vi "HTTPS Server Test with BIO & TCPIP Nodes.vi"() -> ()   [LabVIEW 2013]
uses:
  SSL_Lib/SSL-Lib/Library Paths.ctl
  SSL_Lib/SSL/SSL_Mode.ctl
  SSL_Lib/SSL-Lib/SSL-Lib.lvclass
  SSL_Lib/SSL-Context/SSL-Context.lvclass
  SSL_Lib/SSL/SSL.lvclass
  SSL_Lib/BIO/BIO.lvclass
panel:
  out "Read bytes":string
  out "Numeric":i32
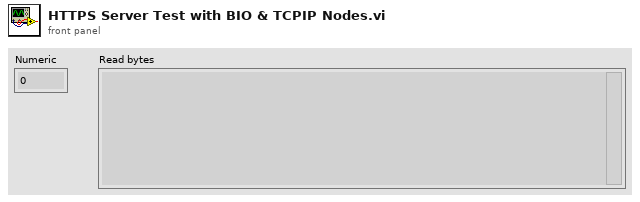
[diagram p1: front panel]
types:
  T1 = typedef "SSL_Lib.lvlib/SSL.lvclass/SSL_Mode.ctl" = i32
  T2 = typedef "SSL_Lib.lvlib/SSL-Lib.lvclass/Library Paths.ctl" = cluster{"SSL Library Path":path, "Crypto Library Path":path}
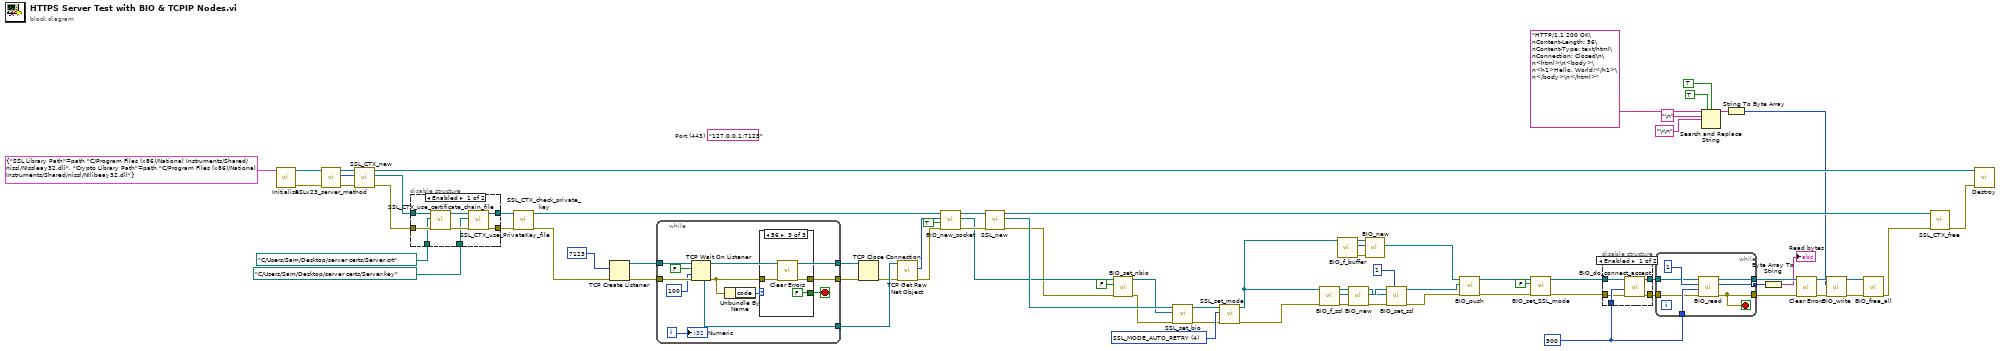
[diagram p0: block diagram]
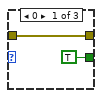
[diagram p3: hidden frame]
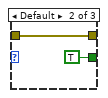
[diagram p4: hidden frame]
diagram:
  w49 = u32 500 ("Timeout (10000ms)")
  (unwired) "127.0.0.1:7123"  # Port (443)
  w63 = T1 4 items=["None"=0, "SSL_MODE_ENABLE_PARTIAL_WRITE"=1, "SSL_MODE_ACCEPT_MOVING_WRITE_BUFFER"=2, "SSL_MODE_AUTO_RETRY"=4, "SSL_MODE_RELEASE_BUFFERS"=16, "SSL_MODE_SEND_FALLBACK_SCSV"=128] ("Mode")
  n1 = call "Initialise.vi"("Library Paths"=T2 {"SSL Library Path"=path "C:/Program Files (x86)/National Instruments/Shared/nissl/NIssleay32.dll", "Crypto Library Path"=path "C:/Program Files (x86)/National Instruments/Shared/nissl/NIlibeay32.dll"}) -> ("error out"=w72:errorcluster, "SSL-Lib out"=w76:refnum<class "SSL-Lib.lvclass">)  [unwired: 9 in]
  n2 = call "SSLv23_server_method.vi"("error in (no error)"=w72, "SSL-Lib in"=w76) -> ("error out"=w70:errorcluster, "*SSL_Method"=w75:u64, "SSL-Lib out"=w74:refnum<class "SSL-Lib.lvclass">)  [unwired: 7 in]
  n3 = call "SSL_CTX_new.vi"("error in (no error)"=w70, "*SSL_Method"=w75, "SSL-Lib in"=w74) -> ("error out"=w69:errorcluster, "SSL-Context out"=w68:refnum<class "SSL-Context.lvclass">, "SSL-Lib out"=w62:refnum<class "SSL-Lib.lvclass">)  [unwired: 6 in]
  n4 = disable-structure shown="Enabled" {
    disable-tunnel: w69 -> [w82 w85]
    disable-tunnel: w68 -> [w81 w86]
    disable-tunnel: [w80 w85] -> w67
    disable-tunnel: [w79 w86] -> w66
    disable-tunnel: path "C:/Users/Sam/Desktop/server certs/Server.crt" -> [w78 _]
    disable-tunnel: path "C:/Users/Sam/Desktop/server certs/Server.key" -> [w77 _]
    frame Enabled {
      n5 = call "SSL_CTX_use_certificate_chain_file.vi"("error in (no error)"=w82, "Certificate Chain File"=w78, "SSL-Context in"=w81) -> ("error out"=w84:errorcluster, "SSL-Context out"=w83:refnum<class "SSL-Context.lvclass">)  [unwired: 7 in]
      n6 = call "SSL_CTX_use_PrivateKey_file.vi"("error in (no error)"=w84, "PrivateKey File"=w77, "SSL-Context in"=w83) -> ("error out"=w80:errorcluster, "SSL-Context out"=w79:refnum<class "SSL-Context.lvclass">)  [unwired: 7 in]
    }
    frame Disabled {
    }
  }
  n7 = call "SSL_CTX_check_private_key.vi"("error in (no error)"=w67, "SSL-Context in"=w66) -> ("error out"=w54:errorcluster, "SSL-Context out"=w43:refnum<class "SSL-Context.lvclass">)  [unwired: 8 in]
  n8 = TCP Create Listener(8:w54, 10:u16 7123 ("port")) -> (0:w60:errorcluster, 3:w59:refnum<k5>)  [unwired: 3 in, 1 out]
  n9 = while {
    tunnel: w60 -> [w97]
    tunnel: w59 -> [w96]
    tunnel: [w95] -> w58
    tunnel: [w91] -> w57
    tunnel: [w94] -> w56
    i -> [w87]
    stop <- w90 stop-if-true
    n10 = TCP Wait On Listener(8:w97, 9:100 ("timeout ms (wait forever: -1)"), 10:FALSE ("resolve remote address (T)"), 11:w96) -> (0:w92:errorcluster, 3:w95:refnum<k5>, 4:w94:refnum<k5>)  [unwired: 2 out]
    n11 = Unbundle By Name(w92) -> ("code"=w93:i32)
    n12 = case shown="56" w93 {
      tunnel: w92 -> [w99 w101 w104]
      tunnel: [w99 w101 w103] -> w91
      tunnel: [TRUE TRUE FALSE] -> w90
      frame 0 {
      }
      frame Default {
      }
      frame 56 {
        n13 = call <vilib>:"Clear Errors.vi"("error in (no error)"=w104) -> ("error out"=w103:errorcluster)  [unwired: 6 in]
      }
    }
    "Numeric" <- w87
  }
  n14 = TCP Close Connection(connection ID=w58, error in (no error)=w57) -> (error out=w55:errorcluster)  [unwired: 1 in, 1 out]
  n15 = call <vilib>:"TCP Get Raw Net Object.vi"("error in (no error)"=w55, "connection ID"=w56) -> ("error out"=w46:errorcluster, "raw net object"=w45:u64)  [unwired: 7 in, 1 out]
  n16 = call "BIO_new_socket.vi"("error in (no error)"=w46, "Close on free? (T)"=TRUE, "fd"=w45, "SSL-Context in"=w43) -> ("error out"=w42:errorcluster, "Socket BIO out"=w39:refnum<class "BIO.lvclass">, "SSL-Context out"=w41:refnum<class "SSL-Context.lvclass">)  [unwired: 5 in]
  n17 = call "SSL_new.vi"("error in (no error)"=w42, "SSL-Context in"=w41) -> ("error out"=w36:errorcluster, "SSL out"=w40:refnum<class "SSL.lvclass">, "SSL-Context out"=w53:refnum<class "SSL-Context.lvclass">)  [unwired: 7 in]
  n18 = call "BIO_set_nbio.vi"("error in (no error)"=w36, "Non-Blocking?"=FALSE, "BIO in"=w39) -> ("error out"=w35:errorcluster, "BIO out"=w37:refnum<class "BIO.lvclass">)  [unwired: 7 in]
  n19 = call "SSL_set_bio.vi"("error in (no error)"=w35, "BIO"=w37, "SSL in"=w40) -> ("error out"=w34:errorcluster, "SSL out"=w38:refnum<class "SSL.lvclass">)  [unwired: 7 in]
  n20 = call "SSL_set_mode.vi"("error in (no error)"=w34, "Mode"=w63, "SSL in"=w38) -> ("error out"=w25:errorcluster, "SSL out"=w18:refnum<class "SSL.lvclass">)  [unwired: 7 in]
  n21 = call "BIO_f_ssl.vi"("error in (no error)"=w25, "SSL-Lib in"=w18) -> ("error out"=w30:errorcluster, "*BIO_Method"=w28:u64, "SSL-Lib out"=w29:refnum<class "SSL.lvclass">)  [unwired: 7 in]
  n22 = call "BIO_f_buffer.vi"("SSL-Lib in"=w18) -> ("error out"=w33:errorcluster, "*BIO_Method"=w31:u64, "SSL-Lib out"=w32:refnum<class "SSL.lvclass">)  [unwired: 8 in]
  n23 = call "BIO_new.vi"("error in (no error)"=w30, "*BIO_method"=w28, "SSL-Lib in"=w29) -> ("error out"=w27:errorcluster, "BIO out"=w26:refnum<class "BIO.lvclass">, "SSL-Lib out"=w24:refnum<class "SSL.lvclass">)  [unwired: 6 in]
  n24 = call "BIO_new.vi"("error in (no error)"=w33, "*BIO_method"=w31, "SSL-Lib in"=w32) -> ("BIO out"=w22:refnum<class "BIO.lvclass">)  [unwired: 6 in, 2 out]
  n25 = call "BIO_set_ssl.vi"("close flag"=1, "error in (no error)"=w27, "SSL in"=w24, "BIO in"=w26) -> ("error out"=w20:errorcluster, "BIO out"=w21:refnum<class "BIO.lvclass">)  [unwired: 6 in]
  n26 = call "BIO_push.vi"("error in (no error)"=w20, "New BIO"=w21, "BIO in"=w22) -> ("error out"=w19:errorcluster, "BIO out"=w16:refnum<class "BIO.lvclass">)  [unwired: 7 in]
  n27 = call "BIO_set_SSL_mode.vi"("error in (no error)"=w19, "Client?"=FALSE, "BIO in"=w16) -> ("error out"=w17:errorcluster, "BIO out"=w15:refnum<class "BIO.lvclass">)  [unwired: 7 in]
  n28 = disable-structure shown="Enabled" {
    disable-tunnel: w15 -> [w109 w111]
    disable-tunnel: w49 -> [w108 _]
    disable-tunnel: [w107 w111] -> w48
    disable-tunnel: [w106 w110] -> w47
    disable-tunnel: w17 -> [w105 w110]
    frame Enabled {
      n29 = call "BIO_do_connect_accept.vi"("error in (no error)"=w105, "Timeout (10000ms)"=w108, "BIO in"=w109) -> ("error out"=w106:errorcluster, "BIO out"=w107:refnum<class "BIO.lvclass">)  [unwired: 7 in]
    }
    frame Disabled {
    }
  }
  n30 = while {
    tunnel: [w117] -> w51 mode=concatenating
    tunnel: w49 -> [w116]
    tunnel: w48 -> [w115]
    tunnel: w47 -> [w114]
    tunnel: [w113] -> w13
    tunnel: [w112] -> w12
    stop <- w112 stop-if-true
    n31 = call "BIO_read.vi"("error in (no error)"=w114, "Timeout (10000ms)"=w116, "bytes to read"=1, "BIO in"=w115) -> ("error out"=w112:errorcluster, "Bytes read"=w117:u8[], "BIO out"=w113:refnum<class "BIO.lvclass">)  [unwired: 5 in]
  }
  n32 = Search and Replace String(replace all?=TRUE ("replace all? (F)"), case sensitive?=TRUE ("ignore case? (F)"), input string="HTTP/1.1 200 OK\nContent-Length: 56\nContent-Type: text/html\nConnection: Closed\n\n<html>\n<body>\n<h1>Hello, World!</h1>\n</body>\n</html>", search string="\n", replace string="\r\n" ("search string")) -> (result string=w5:string)  [unwired: 3 in, 3 out]
  n33 = String To Byte Array(string=w5) -> (unsigned byte array=w9:u8[])
  n34 = Byte Array To String(unsigned byte array=w51) -> (string=→"Read bytes":string)
  n35 = call <vilib>:"Clear Errors.vi"("error in (no error)"=w12) -> ("error out"=w7:errorcluster)  [unwired: 6 in]
  n36 = call "BIO_write.vi"("error in (no error)"=w7, "Bytes to write"=w9, "BIO in"=w13) -> ("error out"=w10:errorcluster, "BIO out"=w11:refnum<class "BIO.lvclass">)  [unwired: 6 in, 1 out]
  n37 = call "BIO_free_all.vi"("error in (no error)"=w10, "BIO in"=w11) -> ("error out"=w50:errorcluster)  [unwired: 9 in]
  n38 = call "SSL_CTX_free.vi"("error in (no error)"=w50, "SSL-Context in"=w53) -> ("error out"=w71:errorcluster)  [unwired: 9 in]
  n39 = call "Destroy.vi"("error in (no error)"=w71, "SSL-Lib in"=w62) -> ()  [unwired: 9 in, 1 out]
